vi "UserPalette-xRainbows.vi"(2 "Teiler":i32=1 min=1 max=5) -> (0 "Array":cluster{u8, u8, u8}[](array[cluster]))   [LabVIEW 2020, in "POLARIS Vision utility.lvlib"]
doc: "User Palette mit Teiler 2**N (1..5)"
uses:
  POLARIS Vision utility.lvlib
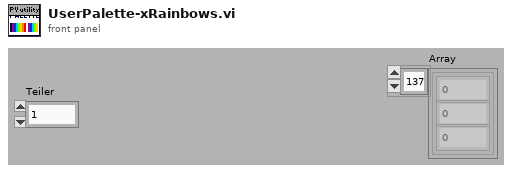
[diagram p1: front panel]
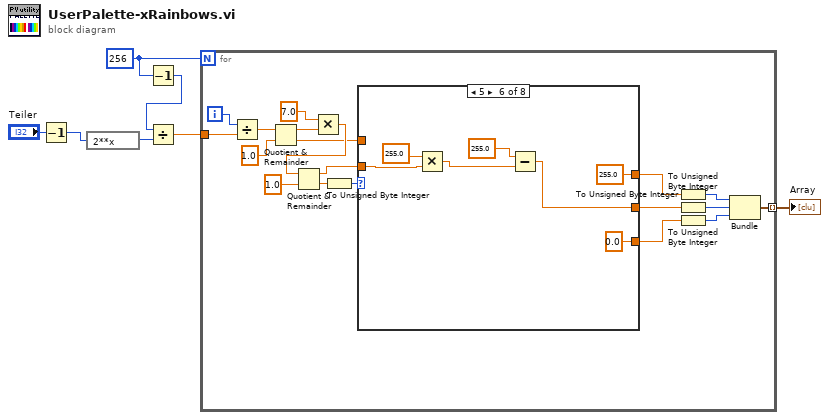
[diagram p0: block diagram]
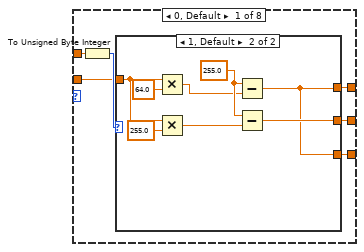
[diagram p2: hidden frame]
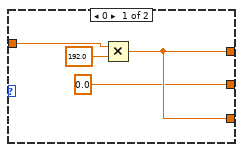
[diagram p3: hidden frame]
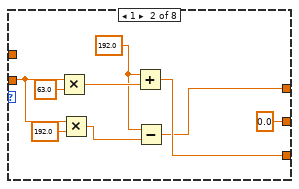
[diagram p4: hidden frame]
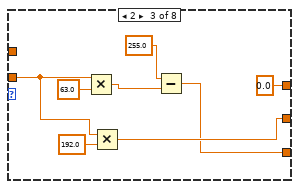
[diagram p5: hidden frame]
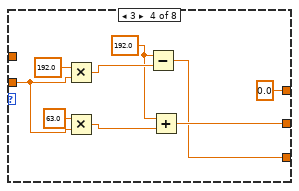
[diagram p6: hidden frame]
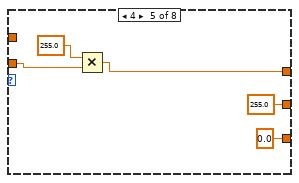
[diagram p7: hidden frame]
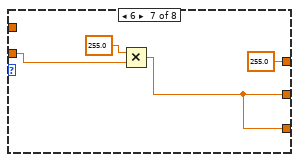
[diagram p8: hidden frame]
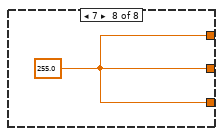
[diagram p9: hidden frame]
diagram:
  w6 = 256
  n1 = Decrement(x="Teiler") -> (x-1=w1:i32)
  n2 = expression code="2**x"(w1) -> (w2:i32)
  n3 = Decrement(x=w6) -> (x-1=w5:i32)
  n4 = Divide(x=w5, y=w2) -> (x/y=w4:dbl)
  n5 = for {
    N: w6 -> [_]
    tunnel: [w26] -> w7 mode=indexing
    tunnel: w4 -> [w21]
    i -> [w22]
    n6 = Divide(x=w22, y=w21) -> (x/y=w20:dbl)
    n7 = Quotient & Remainder(x=w20, y=1.0) -> (x-y*floor(x/y)=w18:dbl, floor(x/y)=w12:dbl)
    n8 = Multiply(x=7.0, y=w18) -> (x*y=w16:dbl)
    n9 = Quotient & Remainder(x=w16, y=1.0) -> (x-y*floor(x/y)=w11:dbl, floor(x/y)=w13:dbl)
    n10 = To Unsigned Byte Integer(number=w13) -> (unsigned 8bit integer=w14:u8)
    n11 = case shown="5" w14 {
      tunnel: w12 -> [w32 _ _ _ _ _ _ _]
      tunnel: w11 -> [w30 w51 w59 w68 w72 w79 w84 _]
      tunnel: [w29 w46 0.0 ("y") 0.0 ("y") w73 255.0 ("y") 255.0 ("y") w87] -> w10
      tunnel: [w27 0.0 ("y") w57 w64 255.0 ("y") w76 w83 w87] -> w9
      tunnel: [w28 w49 w54 w63 0.0 ("y") 0.0 ("y") w83 w87] -> w8
      frame 0, Default {
        n12 = To Unsigned Byte Integer(number=w32) -> (unsigned 8bit integer=w31:u8)
        n13 = case shown="1, Default" w31 {
          tunnel: w30 -> [w35 w42]
          tunnel: [w34 w37] -> w29
          tunnel: [w34 w37] -> w28
          tunnel: [0.0 ("y") w38] -> w27
          frame 0 {
            n14 = Multiply(x=w35, y=192.0) -> (x*y=w34:dbl)
          }
          frame 1, Default {
            w41 = 255.0 ("x")
            n15 = Multiply(x=w42, y=64.0) -> (x*y=w40:dbl)
            n16 = Multiply(x=w42, y=255.0) -> (x*y=w39:dbl)
            n17 = Subtract(x=w41, y=w40) -> (x-y=w37:dbl)
            n18 = Subtract(x=w41, y=w39) -> (x-y=w38:dbl)
          }
        }
      }
      frame 1 {
        w48 = 192.0 ("x")
        n19 = Multiply(x=w51, y=63.0) -> (x*y=w50:dbl)
        n20 = Multiply(x=w51, y=192.0) -> (x*y=w47:dbl)
        n21 = Add(x=w48, y=w50) -> (x+y=w49:dbl)
        n22 = Subtract(x=w48, y=w47) -> (x-y=w46:dbl)
      }
      frame 2 {
        n23 = Multiply(x=w59, y=63.0 ("x")) -> (x*y=w55:dbl)
        n24 = Multiply(x=w59, y=192.0 ("x")) -> (x*y=w57:dbl)
        n25 = Subtract(x=255.0, y=w55) -> (x-y=w54:dbl)
      }
      frame 3 {
        w66 = 192.0 ("x")
        n26 = Multiply(x=192.0, y=w68) -> (x*y=w67:dbl)
        n27 = Multiply(x=63.0, y=w68) -> (x*y=w65:dbl)
        n28 = Subtract(x=w66, y=w67) -> (x-y=w63:dbl)
        n29 = Add(x=w66, y=w65) -> (x+y=w64:dbl)
      }
      frame 4 {
        n30 = Multiply(x=255.0, y=w72) -> (x*y=w73:dbl)
      }
      frame 5 {
        n31 = Multiply(x=255.0 ("y"), y=w79) -> (x*y=w77:dbl)
        n32 = Subtract(x=255.0 ("y"), y=w77) -> (x-y=w76:dbl)
      }
      frame 6 {
        n33 = Multiply(x=255.0 ("y"), y=w84) -> (x*y=w83:dbl)
      }
      frame 7 {
        w87 = 255.0 ("y")
      }
    }
    n34 = To Unsigned Byte Integer(number=w10) -> (unsigned 8bit integer=w23:u8)
    n35 = To Unsigned Byte Integer(number=w9) -> (unsigned 8bit integer=w25:u8)
    n36 = To Unsigned Byte Integer(number=w8) -> (unsigned 8bit integer=w24:u8)
    n37 = Bundle(w23, w25, w24) -> (w26:cluster{u8, u8, u8})  [unwired: 1 in]
  }
  "Array" <- w7
